vi "digital baseband transmission.vi"() -> ()   [LabVIEW 2013]
uses:
  <vilib>/Analysis/2dsp.llb/1D Convolution (DBL).vi
  <vilib>/Analysis/2dsp.llb/Decimate (single shot, DBL).vi
  <vilib>/Analysis/2dsp.llb/Upsample (DBL).vi
  <vilib>/Analysis/NI_AALPro.lvlib
  <vilib>/Analysis/NI_AALBase.lvlib
panel:
  in  "Pluse Shaping Function":enum16{"Sinc", "Rcosine", ""}(ring)
  out "Pluse Shaping":dbl[][](graph)
  out "Baseband":dbl[](graph)
  out "Recovered Bits":i32[](array[numeric])
  in  "stop":bool
  in  "upsampling factor":i32(slide)=1 scale=0.0..100.0
  in  "Sinc Samples":i32=128
  out "Symbol":dbl[](array[numeric])
  in  "Bit":i32[](array[numeric])
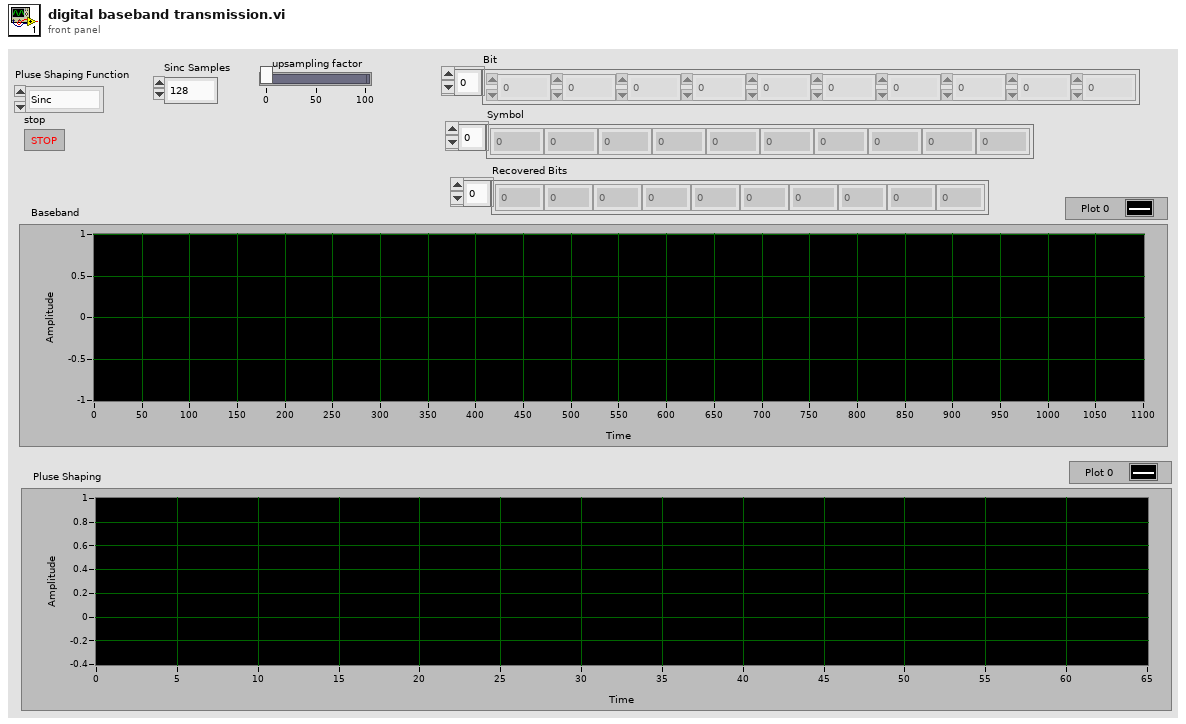
[diagram p1: front panel]
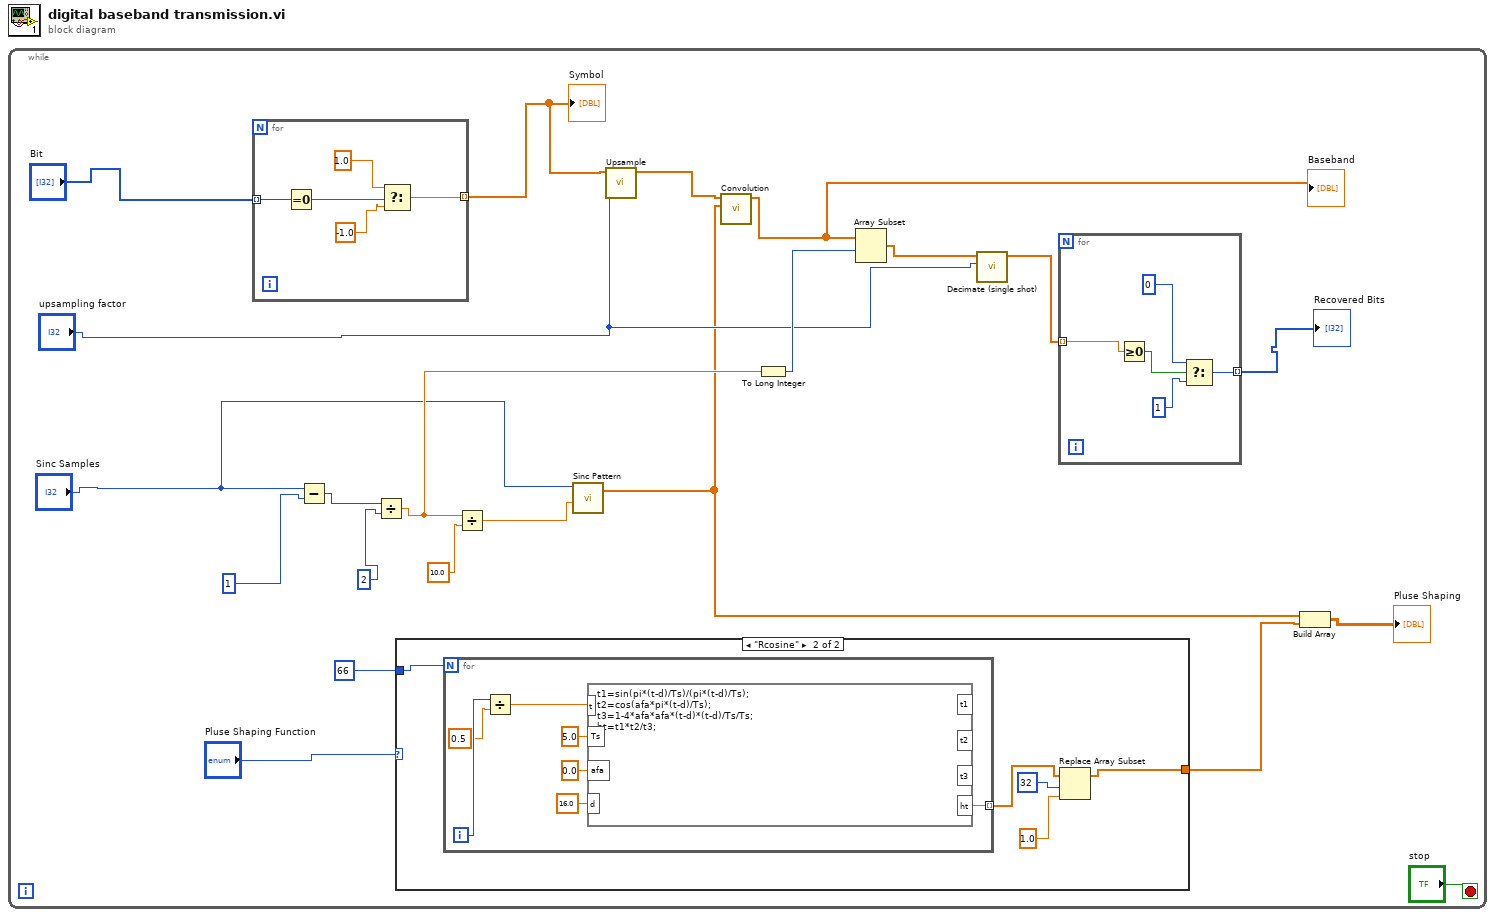
[diagram p0: block diagram]
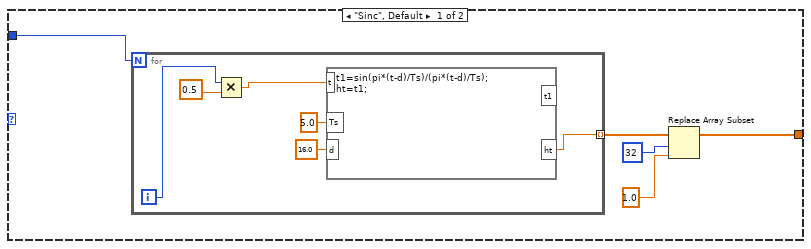
[diagram p2: hidden frame]
diagram:
  n1 = while {
    stop <- "stop" stop-if-true
    n2 = for {
      tunnel: [w52] -> w22 mode=indexing
      tunnel: "Bit" -> [w51] mode=indexing
      n3 = Equal To 0?(x=w51) -> (x = 0?=w55:bool)
      n4 = Select(t=1.0, s=w55, f=-1.0) -> (s? t:f=w52:dbl)
    }
    "Symbol" <- w22
    n5 = Subtract(x="Sinc Samples", y=1) -> (x-y=w17:i32)
    n6 = Divide(x=w17, y=2) -> (x/y=w13:dbl)
    n7 = case shown="\"Rcosine\"" "Pluse Shaping Function" {
      tunnel: 66 -> [w24 w35]
      tunnel: [w23 w34] -> w2
      frame "Sinc", Default {
        n8 = for {
          N: w24 -> [_]
          tunnel: [w28] -> w25 mode=indexing
          i -> [w32]
          n9 = Multiply(x=w32, y=0.5) -> (x*y=w31:dbl)
          n10 = formula code="t1=sin(pi*(t-d)/Ts)/(pi*(t-d)/Ts);\nht=t1;"("t"=w31, "Ts"=5.0 ("input variable"), "d"=16.0 ("input variable")) -> ("ht"=w28:dbl)  [unwired: 1 out]
        }
        n11 = Replace Array Subset "Replace Array Subset"(array=w25, new element=1.0 ("new element/subarray"), index=32) -> (w23:dbl[])
      }
      frame "Rcosine" {
        n12 = for {
          N: w35 -> [_]
          tunnel: [w39] -> w36 mode=indexing
          i -> [w45]
          n13 = Divide(x=w45, y=0.5) -> (x/y=w43:dbl)
          n14 = formula code="t1=sin(pi*(t-d)/Ts)/(pi*(t-d)/Ts);\nt2=cos(afa*pi*(t-d)/Ts);\nt3=1-4*afa*afa*(t-d)*(t-d)/Ts/Ts;\nht=t1*t2/t3;"("t"=w43, "Ts"=5.0 ("input variable"), "afa"=0.0 ("input variable"), "d"=16.0 ("input variable")) -> ("ht"=w39:dbl)  [unwired: 3 out]
        }
        n15 = Replace Array Subset(array=w36, new element=1.0 ("new element/subarray"), index=32) -> (w34:dbl[])
      }
    }
    n16 = Divide(x=w13, y=10.0) -> (x/y=w14:dbl)
    n17 = call <vilib>:"Sinc Pattern.vi"("delay"=w14, "samples"="Sinc Samples") -> ("Sinc Pattern"=w1:dbl[])  [unwired: 2 in, 1 out]
    n18 = call-poly <vilib>:"Upsample.vi"("upsampling factor"="upsampling factor", "X"=w22) -> ("Upsampled Array"=w21:dbl[])  [unwired: 8 in, 1 out]
    n19 = call-poly <vilib>:"Convolution.vi"("Y"=w1, "X"=w21) -> ("X * Y"=w6:dbl[])  [unwired: 8 in, 1 out]
    "Baseband" <- w6
    n20 = To Long Integer(number=w13) -> (32bit integer=w12:i32)
    n21 = Array Subset "Array Subset"(array=w6, index=w12) -> (w20:dbl[])  [unwired: 1 in]
    n22 = call-poly <vilib>:"Decimate (single shot).vi"("decimating factor"="upsampling factor", "X"=w20) -> ("Decimated Array"=w19:dbl[])  [unwired: 8 in, 1 out]
    n23 = for {
      tunnel: w19 -> [w50] mode=indexing
      tunnel: [w46] -> w7 mode=indexing
      n24 = Greater Or Equal To 0?(x=w50) -> (x >= 0?=w49:bool)
      n25 = Select(t=0, s=w49, f=1) -> (s? t:f=w46:i32)
    }
    "Recovered Bits" <- w7
    n26 = Build Array "Build Array"(w1, w2) -> (→"Pluse Shaping":dbl[][])
  }
